vi "位置假-子VI1.vi"() -> (20 "8":string="0", 21 "9":string="0", 22 "10":string="0", 23 "11":string="0", 24 "12":string="0", 25 "13":string="0", 26 "14":string="0", 27 "15":string="0")   [LabVIEW 2014]
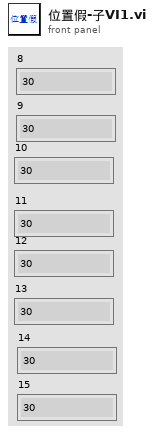
[diagram p1: front panel]
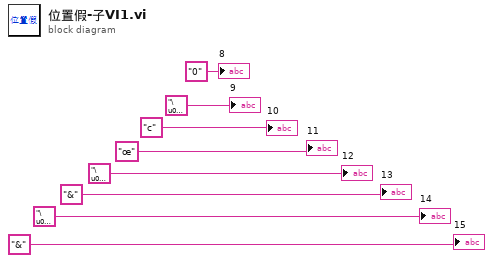
[diagram p0: block diagram]
diagram:
  "8" <- "0"
  "9" <- "\u0000"
  "10" <- "c"
  "11" <- "œ"
  "12" <- "\u0002"
  "13" <- "&"
  "14" <- "\u0002"
  "15" <- "&"
